vi "Write ini file.vi"(4 "Write All?":bool, 6 "Selected Plate":i32, 7 "file path (use dialog)":path, 8 "error in":errorcluster, 9 "Standalone?":bool, 10 "INI Data":T2(array[cluster]), 11 "Config File Ref Num":T1) -> (0 "error out":errorcluster, 3 "refnum out":T1)   [LabVIEW 2017]
uses:
  <vilib>/Utility/config.llb/Config Data RefNum.ctl
  <vilib>/Utility/config.llb/Write Key (String).vi
  <vilib>/Utility/config.llb/NI_LVConfig.lvlib
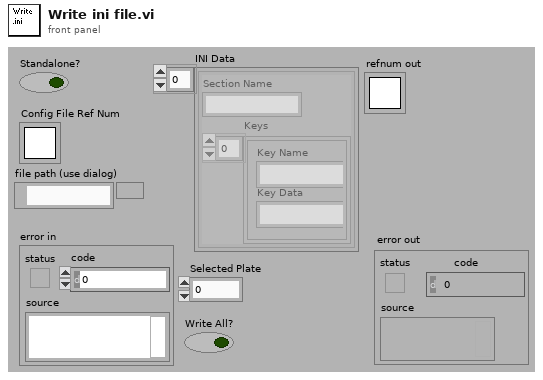
[diagram p1: front panel]
types:
  T1 = typedef "NI_LVConfig.lvlib/Config Data RefNum.ctl" = refnum<k1>
  T2 = cluster{"Section Name":string, "Keys":cluster{"Key Name":string, "Key Data":string}[]}[]
  T3 = cluster{"Section Name":string, "Keys":cluster{"Key Name":string, "Key Data":string}[]}
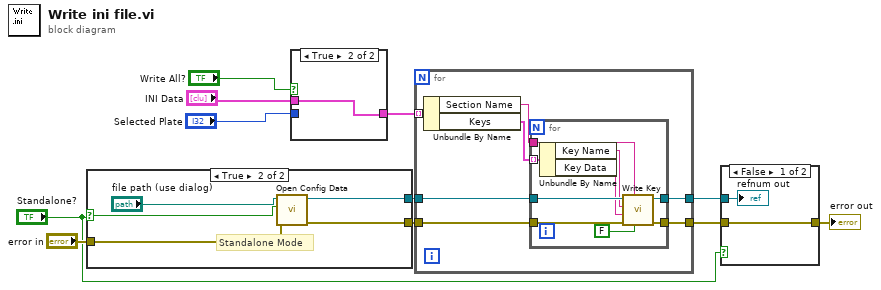
[diagram p0: block diagram]
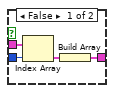
[diagram p2: hidden frame]
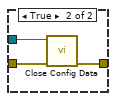
[diagram p3: hidden frame]
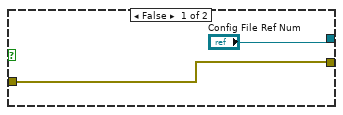
[diagram p4: hidden frame]
diagram:
  n1 = case shown="True" "Standalone?" {
    selector: "Standalone?" -> [_ w15]
    tunnel: [w13 w18] -> w11
    tunnel: ["Config File Ref Num" w17] -> w10
    tunnel: "error in" -> [w13 w14]
    frame False {
    }
    frame True {
      # "Standalone Mode"
      n2 = call <vilib>:"Open Config Data.vi"("error in (no error)"=w14, "create file if necessary (T)"=w15, "configuration file path"="file path (use dialog)") -> ("error out"=w18:errorcluster, "refnum"=w17:T1)  [unwired: 6 in, 1 out]
    }
  }
  n3 = case shown="True" "Write All?" {
    tunnel: "INI Data" -> [w22 w23]
    tunnel: [w19 w23] -> w3
    tunnel: "Selected Plate" -> [w20 _]
    frame False {
      n4 = Index Array(array=w22, index=w20) -> (element=w21:T3)
      n5 = Build Array(w21) -> (w19:T2)
    }
    frame True {
    }
  }
  n6 = for {
    tunnel: w11 -> [w30]
    tunnel: w10 -> [w29]
    tunnel: w3 -> [w28] mode=indexing
    tunnel: [w25] -> w8
    tunnel: [w24] -> w9
    n7 = Unbundle By Name(w28) -> ("Section Name"=w27:string, "Keys"=w26:cluster{"Key Name":string, "Key Data":string}[])
    n8 = for {
      tunnel: w30 -> [w39]
      tunnel: w29 -> [w38]
      tunnel: w27 -> [w37]
      tunnel: w26 -> [w34] mode=indexing
      tunnel: [w36] -> w25
      tunnel: [w35] -> w24
      n9 = Unbundle By Name(w34) -> ("Key Name"=w33:string, "Key Data"=w32:string)
      n10 = call-poly <vilib>:"Write Key.vi"("write raw string? (F)"=FALSE, "section"=w37, "error in (no error)"=w39, "value"=w32, "key"=w33, "refnum"=w38) -> ("error out"=w35:errorcluster, "refnum out"=w36:T1)  [unwired: 4 out]
    }
  }
  n11 = case shown="False" "Standalone?" {
    tunnel: w9 -> [w41 w44]
    tunnel: w8 -> [w40 w43]
    tunnel: [w41 w42] -> w7
    frame False {
      "refnum out" <- w40
    }
    frame True {
      n12 = call <vilib>:"Close Config Data.vi"("error in (no error)"=w44, "refnum"=w43) -> ("error out"=w42:errorcluster)  [unwired: 1 in, 8 out]
    }
  }
  "error out" <- w7
